vi "Three part tester.vi"() -> ()   [LabVIEW 2009]
uses:
  <vilib>/Instr/_visa.llb/VISA Configure Serial Port (Instr).vi
panel:
  out "decimal integer string 3":string
  out "number 3":u8 format="%b"
  in  "Foot Pedal":bool
  in  "Orange Guitar LED":bool
  in  "Blue Guitar LED":bool
  in  "Red Guitar LED":bool
  in  "Green Guitar LED":bool
  in  "Yellow Guitar LED":bool
  in  "GreenDrum":bool
  out "Guitar Cluster":T1
  out "Bass Cluster":T2
  out "Drum Cluster":T3
  in  "Stop":bool
  out "decimal integer string 2":string
  out "number 2":u8 format="%b"
  in  "Orange Bass LED":bool
  in  "Yellow Bass LED":bool
  in  "Green Bass LED":bool
  in  "Red Bass LED":bool
  in  "Blue Bass LED":bool
  in  "Red Drum":bool
  in  "VISA resource name":refnum<visa-resource-name>
  out "number":u8 format="%b"
  out "decimal integer string":string
  in  "Yellow Drum":bool
  in  "Blue Drum":bool
  # "Drums"
  # "Bass"
  # "Guitar"
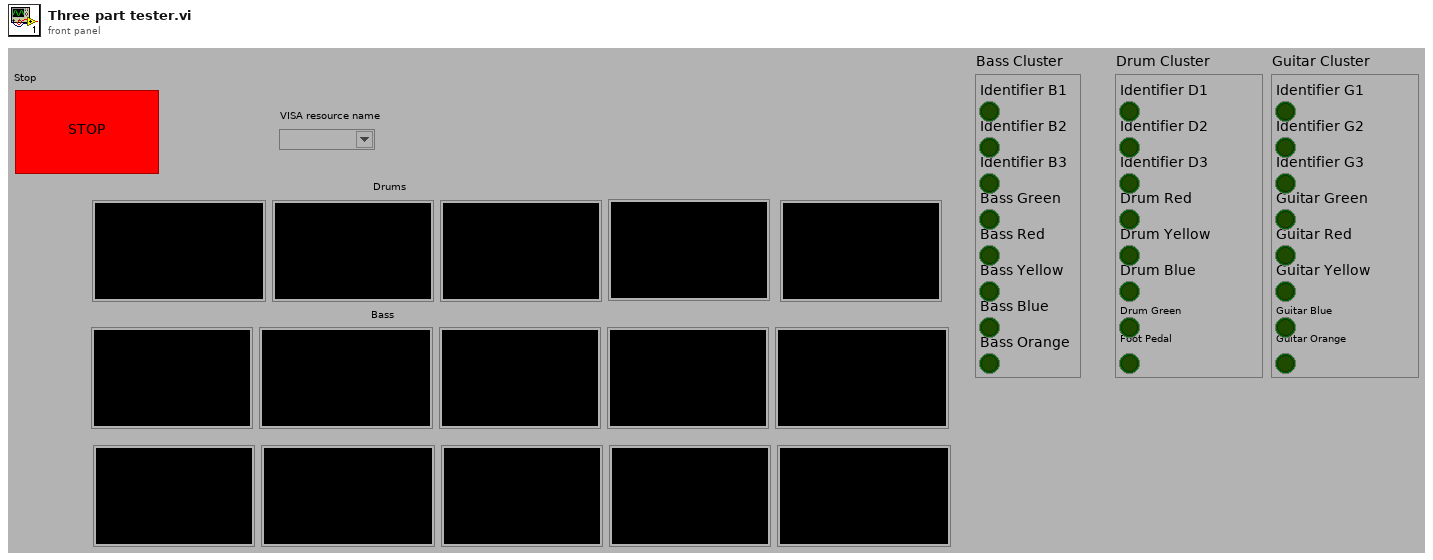
[diagram p1: front panel]
types:
  T1 = cluster{"Identifier G1":bool, "Identifier G2":bool, "Identifier G3":bool, "Guitar Green":bool, "Guitar Red":bool, "Guitar Yellow":bool, "Guitar Blue":bool, "Guitar Orange":bool}
  T2 = cluster{"Identifier B1":bool, "Identifier B2":bool, "Identifier B3":bool, "Bass Green":bool, "Bass Red":bool, "Bass Yellow":bool, "Bass Blue ":bool, "Bass Orange":bool}
  T3 = cluster{"Identifier D1":bool, "Identifier D2":bool, "Identifier D3":bool, "Drum Red":bool, "Drum Yellow":bool, "Drum Blue":bool, "Drum Green":bool, "Foot Pedal":bool}
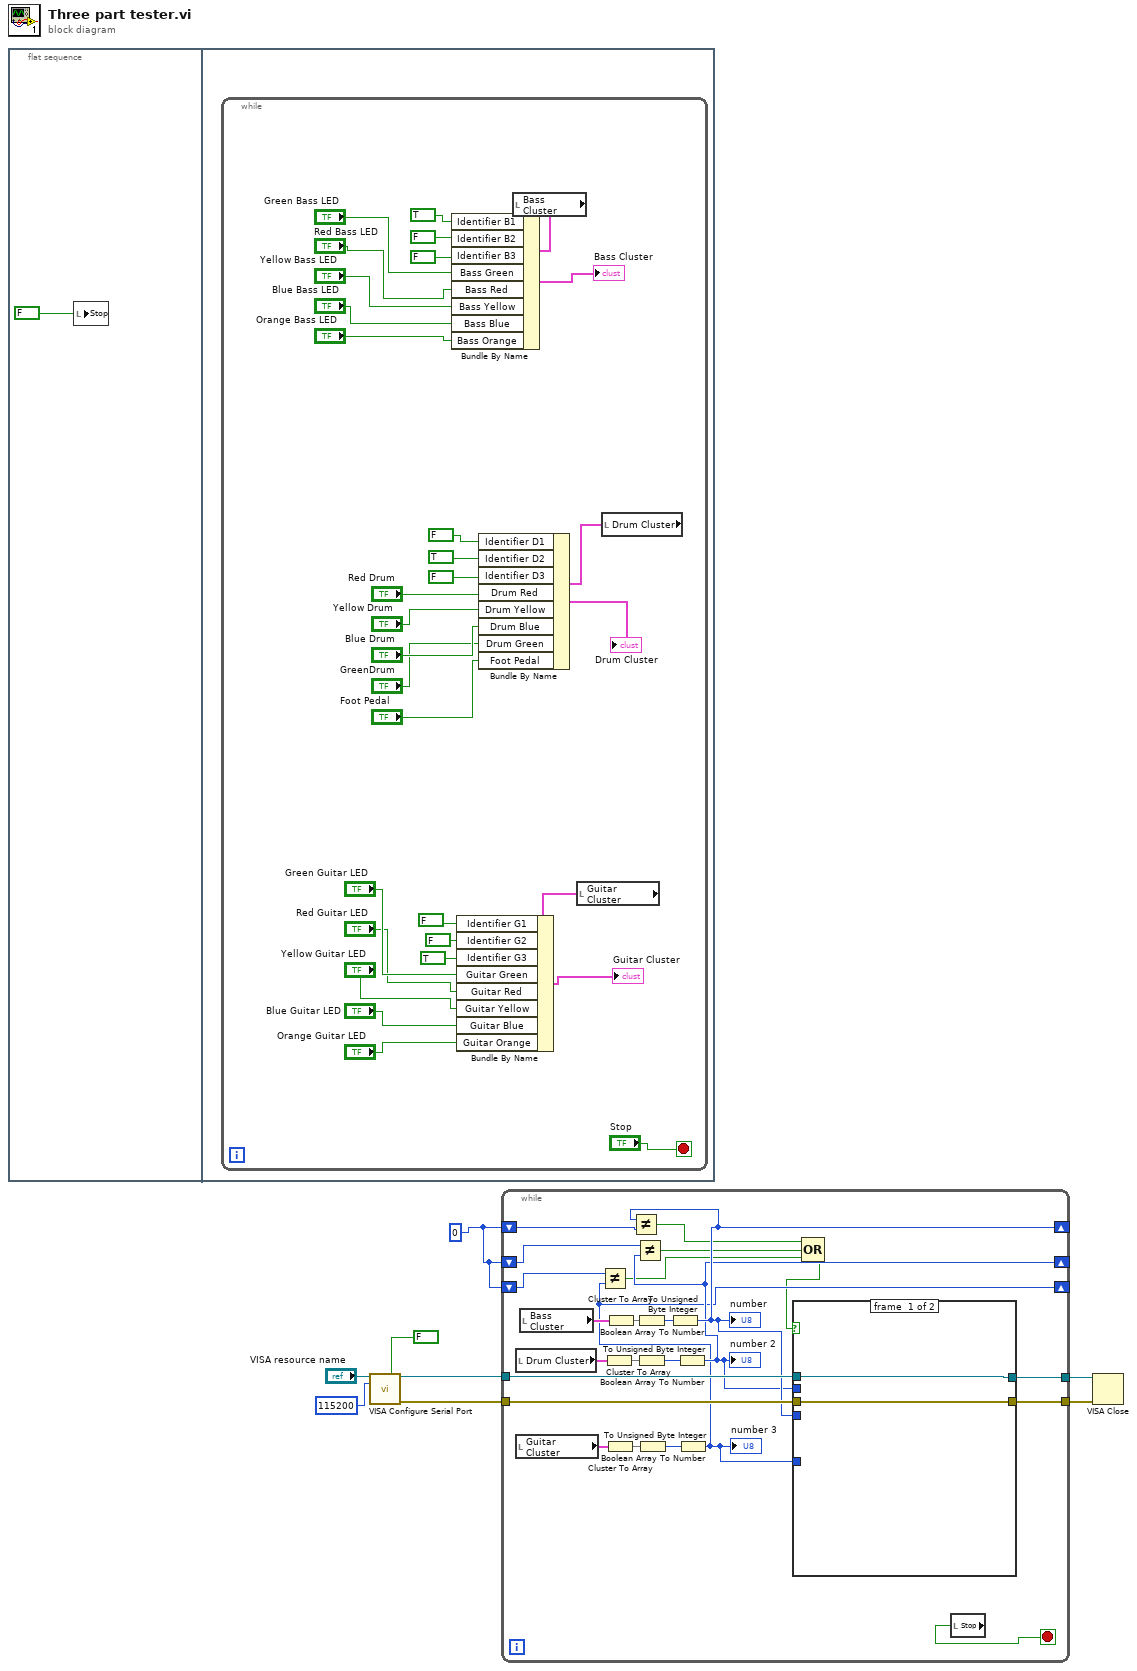
[diagram p0: block diagram]
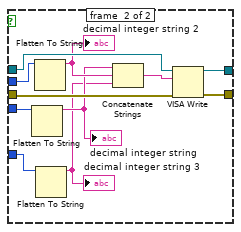
[diagram p2: hidden frame]
diagram:
  w1 = u8 0
  n1 = flat-sequence {
    frame #0 {
      n2 = local write "Stop"(FALSE ("Stop 2")) -> ()
    }
    frame #1 {
      n3 = while {
        stop <- "Stop" stop-if-true
        n4 = local read "Bass Cluster"() -> (w39:T2)
        n5 = Bundle By Name(cluster=w39, "Identifier B1"=TRUE, "Identifier B2"=FALSE ("element"), "Identifier B3"=FALSE ("element"), "Bass Green"="Green Bass LED", "Bass Red"="Red Bass LED", "Bass Yellow"="Yellow Bass LED", "Bass Blue"="Blue Bass LED", "Bass Orange"="Orange Bass LED") -> (→"Bass Cluster":T2)
        n6 = local read "Guitar Cluster"() -> (w27:T1)
        n7 = Bundle By Name(cluster=w27, "Identifier G1"=FALSE ("element"), "Identifier G2"=FALSE ("element"), "Identifier G3"=TRUE ("element"), "Guitar Green"="Green Guitar LED", "Guitar Red"="Red Guitar LED", "Guitar Yellow"="Yellow Guitar LED", "Guitar Blue"="Blue Guitar LED", "Guitar Orange"="Orange Guitar LED") -> (→"Guitar Cluster":T1)
        n8 = local read "Drum Cluster"() -> (w32:T3)
        n9 = Bundle By Name(cluster=w32, "Identifier D1"=FALSE, "Identifier D2"=TRUE ("element"), "Identifier D3"=FALSE ("element"), "Drum Red"="Red Drum", "Drum Yellow"="Yellow Drum", "Drum Blue"="Blue Drum", "Drum Green"="GreenDrum", "Foot Pedal"="Foot Pedal") -> (→"Drum Cluster":T3)
      }
    }
  }
  n10 = call-poly "VISA Configure Serial Port"("VISA resource name"="VISA resource name", "Enable Termination\nChar (T)"=FALSE ("Enable Termination\nChar (T)"), "baud rate (9600)"=u32 115200) -> ("VISA resource name out"=w8:refnum<visa-resource-name>, "error out"=w3:errorcluster)  [unwired: 11 in]
  n11 = while {
    tunnel: w8 -> [w64]
    tunnel: [w63] -> w7
    tunnel: w3 -> [w62]
    tunnel: [w61] -> w2
    shift-right: [w53] -> _
    shift-left: w1 -> [w52]
    shift-right: [w51] -> _
    shift-left: w1 -> [w50]
    shift-right: [w45] -> _
    shift-left: w1 -> [w46]
    stop <- w56 stop-if-true
    n12 = local read "Drum Cluster"() -> (w58:T3)
    n13 = local read "Guitar Cluster"() -> (w48:T1)
    n14 = local read "Bass Cluster"() -> (w57:T2)
    n15 = Cluster To Array(cluster=w58) -> (array=w59:bool[])
    n16 = Cluster To Array(cluster=w48) -> (array=w47:bool[])
    n17 = Cluster To Array(cluster=w57) -> (array=w60:bool[])
    n18 = Boolean Array To Number(Boolean array=w60) -> (number=w55:u32)
    n19 = Boolean Array To Number(Boolean array=w59) -> (number=w54:u32)
    n20 = Boolean Array To Number(Boolean array=w47) -> (number=w49:u32)
    n21 = To Unsigned Byte Integer(number=w55) -> (unsigned 8bit integer=w53:u8)
    "number" <- w53
    n22 = Not Equal?(x=w53, y=w52) -> (x != y?=w43:bool)
    n23 = To Unsigned Byte Integer(number=w54) -> (unsigned 8bit integer=w51:u8)
    "number 2" <- w51
    n24 = Not Equal?(x=w50, y=w51) -> (x != y?=w42:bool)
    n25 = To Unsigned Byte Integer(number=w49) -> (unsigned 8bit integer=w45:u8)
    "number 3" <- w45
    n26 = Not Equal?(x=w46, y=w45) -> (x != y?=w41:bool)
    n27 = Compound Arithmetic op=OR(w43, w42, w41) -> (w44:bool)
    n28 = case shown="True" w44 {
      tunnel: w64 -> [w66 w77]
      tunnel: [w66 w76] -> w63
      tunnel: w53 -> [_ w70]
      tunnel: w62 -> [w65 w75]
      tunnel: [w65 w74] -> w61
      tunnel: w51 -> [_ w72]
      tunnel: w45 -> [_ w67]
      frame #0 {
      }
      frame #1 {
        n29 = Flatten To String(anything=w70) -> (data string=w69:string)  [unwired: 3 in, 2 out]
        "decimal integer string" <- w69
        n30 = Flatten To String(anything=w72) -> (data string=w71:string)  [unwired: 3 in, 2 out]
        "decimal integer string 2" <- w71
        n31 = Flatten To String(anything=w67) -> (data string=w68:string)  [unwired: 3 in, 2 out]
        "decimal integer string 3" <- w68
        n32 = Concatenate Strings(w69, w71, w68) -> (w73:string)
        n33 = VISA Write(VISA resource name=w77, write buffer=w73, error in (no error)=w75) -> (VISA resource name out=w76:refnum<visa-resource-name>, error out=w74:errorcluster)  [unwired: 1 out]
      }
    }
    n34 = local read "Stop"() -> (w56:bool)
  }
  n35 = VISA Close(VISA resource name=w7, error in (no error)=w2) -> ()  [unwired: 1 out]
